vi "path gen.vi"(8 "error in":errorcluster, 11 "Calling VI":refnum<vi>) -> (0 "error out":errorcluster, 2 "basename":string, 3 "output folder":path)   [LabVIEW 2020]
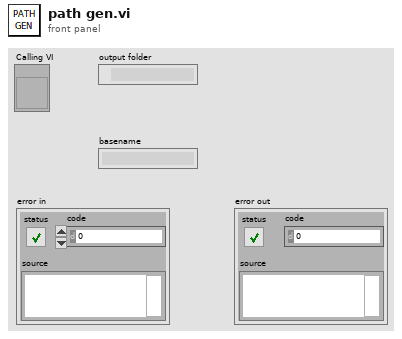
[diagram p1: front panel]
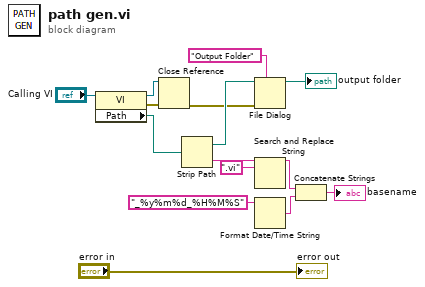
[diagram p0: block diagram]
diagram:
  n1 = property class="VI"(reference="Calling VI") -> (reference out=w3:refnum<vi>, error out=w4:errorcluster, "Path"=w5:path)  [unwired: 1 in]
  n2 = Close Reference(reference=w3, error in (no error)=w4) -> (error out=w2:errorcluster)
  n3 = Strip Path(path=w5) -> (stripped path=w8:path, name=w7:string)
  n4 = File Dialog(7:"Output Folder" ("prompt"), 8:w2, 11:w8) -> (3:→"output folder":path)  [unwired: 4 in, 3 out]
  n5 = Search and Replace String(input string=w7, search string=".vi") -> (result string=w13:string)  [unwired: 6 in, 3 out]
  n6 = Format Date/Time String(time format string (%c)="_%y%m%d_%H%M%S") -> (date/time string=w14:string)  [unwired: 2 in]
  n7 = Concatenate Strings(w13, w14) -> (→"basename":string)
  "error out" <- "error in"
